vi "Two Processes.vi"() -> ()   [LabVIEW 2010]
doc: "This VI demonstrates two processes which cannot run in parallel is their current configuration."
panel:
  out "Input Data":dbl(graph)
  in  "stop":bool
  out "Value > 0?":bool
  out "Current Time":timestamp format="%<%I:%M:%S %p\n%x>T"
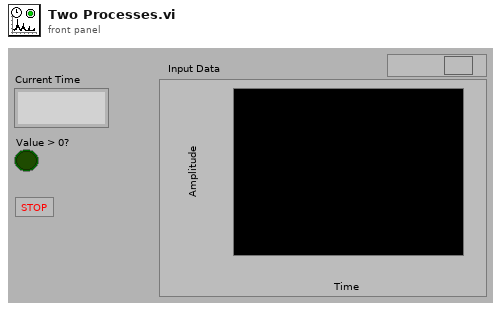
[diagram p1: front panel]
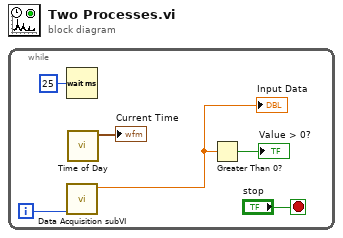
[diagram p0: block diagram]
diagram:
  n1 = while {
    i -> [w3]
    stop <- "stop" stop-if-true
    n2 = Wait (ms)(milliseconds to wait=u32 25) -> ()  [unwired: 1 out]
    n3 = call "Data Acquisition subVI.vi"("Numeric in"=w3) -> ("Numeric out"=w5:dbl)  [unwired: 10 in]
    "Input Data" <- w5
    n4 = call "Time of Day.vi"() -> ("current time"=→"Current Time":timestamp)  [unwired: 11 in]
    n5 = Greater Than 0?(x=w5) -> (x > 0?=→"Value > 0?":bool)
  }
